vi "JOYSTICK.vi"() -> ()   [LabVIEW 2016]
uses:
  <vilib>/Math Plots/2D Math Plots/2D Compass/2D Compass XCtrl/2D Compass.xctl
  <vilib>/LabVIEW Interface for Arduino/Type Defs/Board Type.ctl
  <vilib>/LabVIEW Interface for Arduino/Type Defs/Connection Type.ctl
  <vilib>/Math Plots/2D Math Plots/2D Compass/2D Compass Datatype/Public/Plot Helper (Vector).vi
  <vilib>/Math Plots/2D Math Plots/2D Compass/2D Compass Datatype/2D Compass Datatype.lvclass
  <vilib>/LabVIEW Interface for Arduino/LabVIEW Interface for Arduino.lvlib
panel:
  out "2D Compass":refnum<class "2D Plot Datatype.lvclass">[](xcontrol)
  in  "stop":bool
  out "Magnitud":dbl
  out "Angulo Grados":dbl
  out "Angulo Rad":dbl
  out "SW":dbl
  out "Y Axis":dbl(knob) scale=0.0..5.0
  out "X Axis":dbl(knob) scale=0.0..5.0
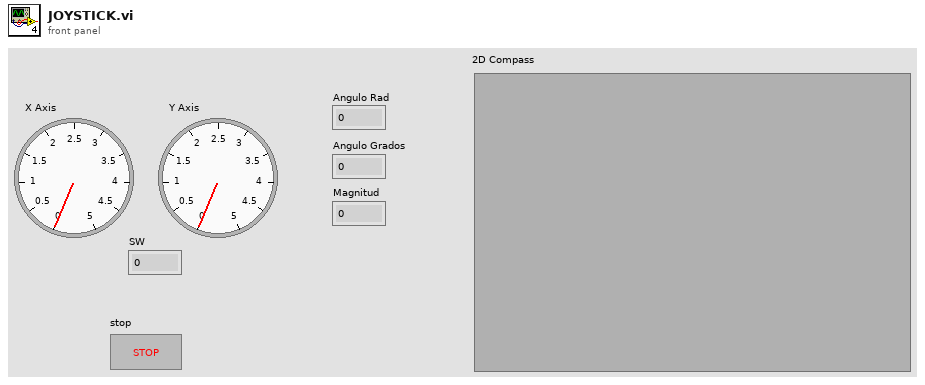
[diagram p1: front panel]
types:
  T1 = typedef "LabVIEW Interface for Arduino.lvlib/Connection Type.ctl" = enum8{"USB / Serial", "XBEE", "BlueSmirf (Bluetooth)"}
  T2 = typedef "LabVIEW Interface for Arduino.lvlib/Board Type.ctl" = enum16{"Uno", "Dimuelanove w/Atmega 328", "Mega 2560"}
  T3 = typedef "LabVIEW Interface for Arduino.lvlib/Arduino Resource.ctl" = cluster{"VISA resource":refnum<visa-resource-name>, "Board Type":T2, "Connection Type":enum8{"USB / Serial"}, "Bytes Per Packet (15)":u8}
  T4 = cluster{"Horizontal Axis Pin":dbl, "Vertical Axis Pin":dbl, "Select Pin":dbl}
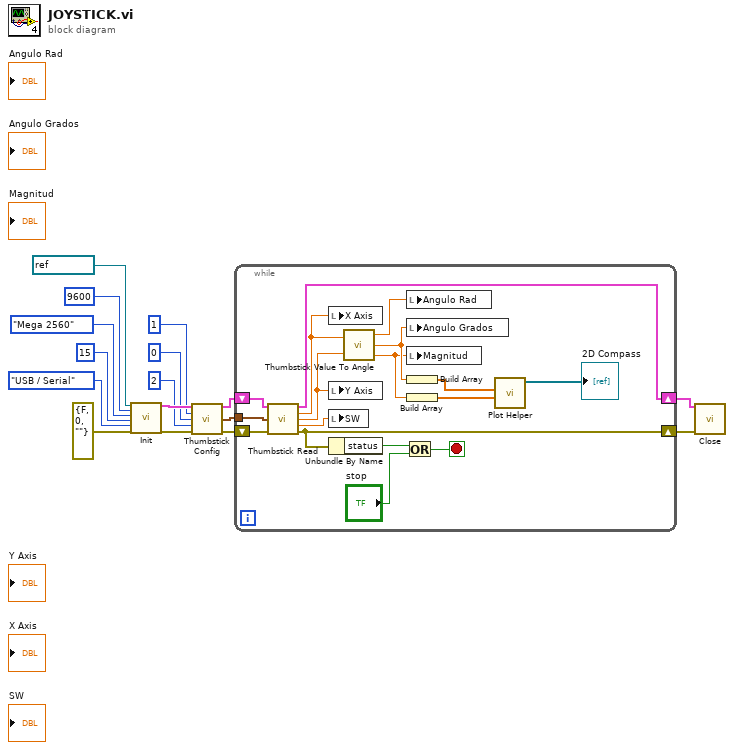
[diagram p0: block diagram]
diagram:
  n1 = call <vilib>:"Init.vi"("VISA resource"=refnum<visa-resource-name> "COM6", "Baud Rate (115200)"=u32 9600, "Board Type (Uno)"=Board_Type."Mega 2560", "Bytes Per Packet (15)"=u32 15, "Connection Type (USB/Serial)"=Connection_Type."USB / Serial", "error in"=errorcluster {"status"=FALSE, "code"=0, "source"=""}) -> ("Arduino Resource"=w16:T3, "error out"=w15:errorcluster)  [unwired: 12 in]
  n2 = call <vilib>:"Thumbstick Config.vi"("Arduino Resource"=w16, "Horizontal Axis AI Pin"=u8 1, "Vertical Axis AI Pin"=u8 0, "Select DI Pin"=u8 2, "error in"=w15) -> ("Arduino Resource"=w5:T3, "Thumbstick Data"=w3:T4, "error out"=w4:errorcluster)  [unwired: 8 in]
  n3 = while {
    tunnel: w3 -> [w31]
    shift-right: [w17] -> w1
    shift-left: w4 -> [w32]
    shift-right: [w18] -> w2
    shift-left: w5 -> [w33]
    stop <- w28 stop-if-true
    n4 = call <vilib>:"Thumbstick Read.vi"("Arduino Resource"=w33, "Thumbstick Data"=w31, "error in"=w32) -> ("Arduino Resource"=w18:T3, "Horizontal Axis"=w25:dbl, "Vertical Axis"=w24:dbl, "Select (Active Low)"=w30:dbl, "error out"=w17:errorcluster)  [unwired: 8 in]
    n5 = local write "X Axis"(w25) -> ()
    n6 = local write "Y Axis"(w24) -> ()
    n7 = local write "SW"(w30) -> ()
    n8 = Unbundle By Name(w17) -> ("status"=w29:bool)
    n9 = call <vilib>:"Thumbstick Value To Angle.vi"("Vertical Axis"=w24, "Horizontal Axis"=w25) -> ("Magnitude"=w20:dbl, "Degrees"=w21:dbl, "Radians"=w23:dbl)
    n10 = Or(x=w29, y="stop") -> (x .or. y?=w28:bool)
    n11 = local write "Angulo Rad"(w23) -> ()
    n12 = local write "Angulo Grados"(w21) -> ()
    n13 = local write "Magnitud"(w20) -> ()
    n14 = Build Array(w21) -> (w22:dbl[])
    n15 = Build Array(w20) -> (w19:dbl[])
    n16 = call-poly <vilib>:"Plot Helper.vi"("radius vector"=w19, "theta vector"=w22) -> ("2D Plot Class Obj Array out"=→"2D Compass":refnum<class "2D Plot Datatype.lvclass">[])  [unwired: 2 in, 7 out]
  }
  n17 = call <vilib>:"Close.vi"("Arduino Resource"=w2, "error in"=w1) -> ()  [unwired: 13 in, 1 out]
